vi "Add Vector Arrow to 3D Plot.vi"(6 "% of Shaft to Tip":dbl=0.8, 8 "Scale %":dbl=1.0, 9 "Unit Vector?":bool, 10 "Vector Color":u32(colorbox)=16879, 11 "Vector":dbl[](array[numeric])=[1.0, 0.0, 0.0]) -> (3 "Vector Arrow Object":refnum<vi>)   [LabVIEW 2010]
uses:
  <vilib>/picture/3D Picture Control/NI_3D Picture Control.lvlib
panel:
  out "3D Picture":refnum<vi>(3d-picture)
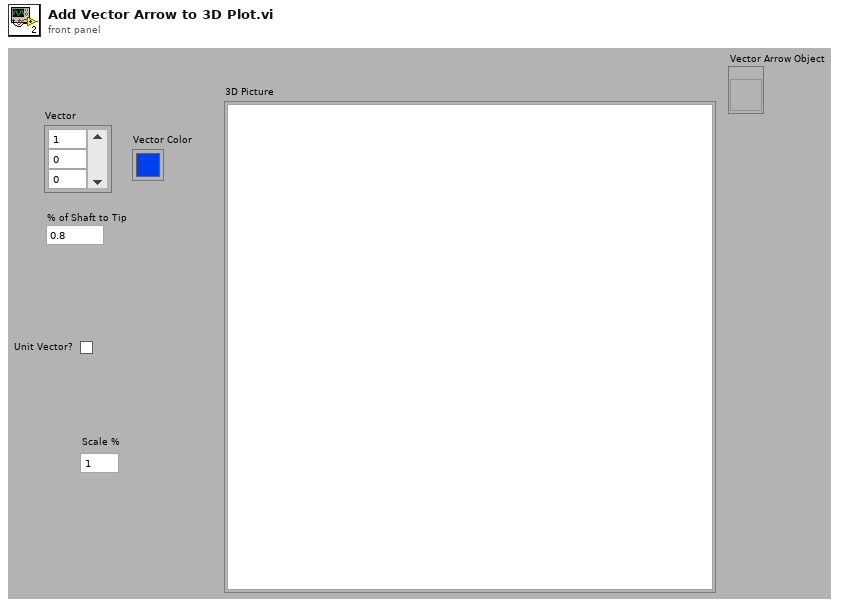
[diagram p1: front panel]
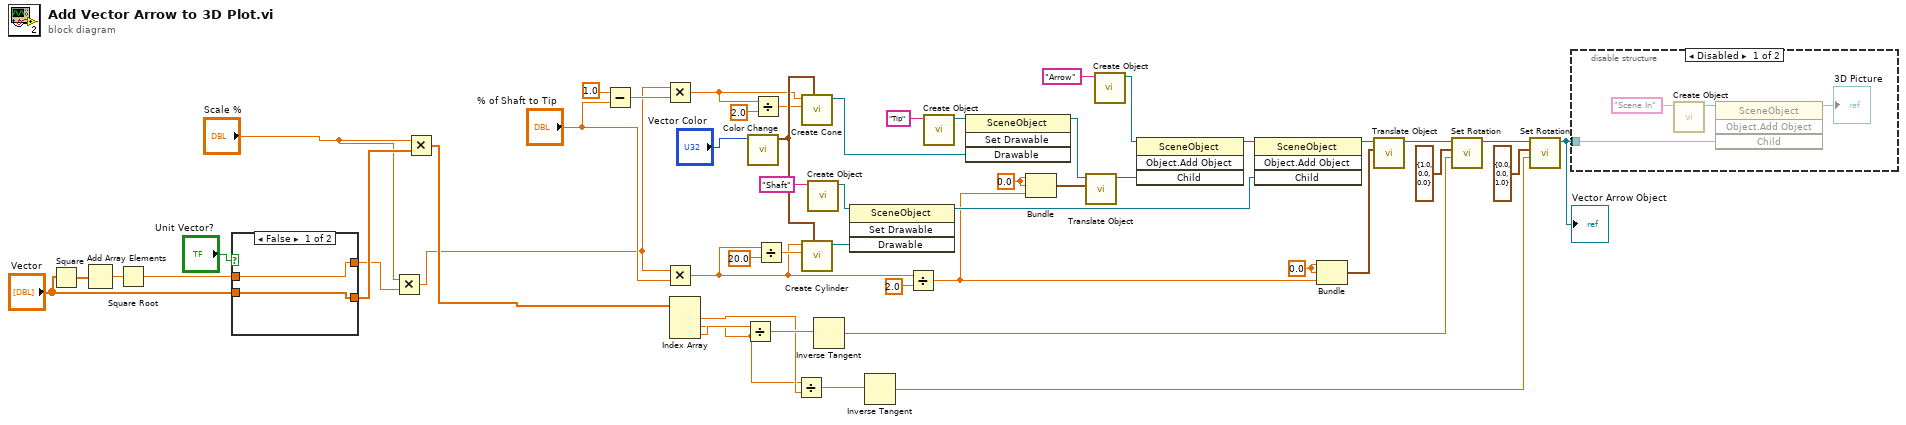
[diagram p0: block diagram]
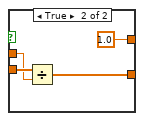
[diagram p2: hidden frame]
diagram:
  w23 = 0.0 ("x")
  w26 = 0.0 ("x")
  n1 = Square(x="Vector") -> (x^2=w20:dbl[])
  n2 = Add Array Elements(numeric array=w20) -> (sum=w19:dbl)
  n3 = Square Root(x=w19) -> (sqrt(x)=w16:dbl)
  n4 = case shown="False" "Unit Vector?" {
    tunnel: "Vector" -> [w53 w58]
    tunnel: w16 -> [w54 w57]
    tunnel: [w54 1.0] -> w3
    tunnel: [w53 w55] -> w5
    frame False {
    }
    frame True {
      n5 = Divide(x=w58, y=w57) -> (x/y=w55:dbl[])
    }
  }
  n6 = Multiply(x="Scale %", y=w3) -> (x*y=w1:dbl)
  n7 = Multiply(x="Scale %", y=w5) -> (x*y=w4:dbl[])
  n8 = Subtract(x=1.0, y="% of Shaft to Tip") -> (x-y=w38:dbl)
  n9 = Multiply(x=w1, y=w38) -> (x*y=w29:dbl)
  n10 = Multiply(x=w1, y="% of Shaft to Tip") -> (x*y=w30:dbl)
  n11 = Index Array(array=w4) -> (element #1=w8:dbl, element #2=w7:dbl, element #3=w12:dbl)  [unwired: 3 in]
  n12 = Divide(x=w12, y=w7) -> (x/y=w11:dbl)
  n13 = call <vilib>:"Color Change.vi"("Color"="Vector Color") -> ("RGBA"=w41:cluster{"R":sgl, "G":sgl, "B":sgl, "A":sgl})  [unwired: 10 in]
  n14 = Divide(x=w29, y=2.0) -> (x/y=w27:dbl)
  n15 = Divide(x=w30, y=20.0) -> (x/y=w31:dbl)
  n16 = Divide(x=w7, y=w8) -> (x/y=w9:dbl)
  n17 = call <vilib>:"Create Cone.vi"("Color"=w41, "Radius"=w27, "Height"=w29) -> ("New Cone Refnum"=w47:refnum<vi>)  [unwired: 7 in, 1 out]
  n18 = call <vilib>:"Create Cylinder.vi"("Color"=w41, "Radius"=w31, "Height"=w30) -> ("New Cylinder Refnum"=w46:refnum<vi>)  [unwired: 7 in, 1 out]
  n19 = call <vilib>:"Create Object.vi"("Name"="Shaft") -> ("Scene:New Object"=w44:refnum<vi>)  [unwired: 1 in, 9 out]
  n20 = Inverse Tangent(1:w11) -> (0:w10:dbl)
  n21 = invoke class="SceneObject" method="Set Drawable"(reference=w44, "Drawable"=w46) -> (reference out=w43:refnum<vi>)  [unwired: 2 in, 3 out]
  n22 = Inverse Tangent(1:w9) -> (0:w6:dbl)
  n23 = Divide(x=w30, y=2.0) -> (x/y=w21:dbl)
  n24 = call <vilib>:"Create Object.vi"("Name"="Tip") -> ("Scene:New Object"=w48:refnum<vi>)  [unwired: 1 in, 9 out]
  n25 = invoke class="SceneObject" method="Set Drawable"(reference=w48, "Drawable"=w47) -> (reference out=w37:refnum<vi>)  [unwired: 2 in, 3 out]
  n26 = Bundle("x"=w26, "x"=w26, w21) -> (w34:cluster{"x":dbl, "x":dbl, dbl})  [unwired: 1 in]
  n27 = call <vilib>:"Translate Object.vi"("Translation"=w34, "Scene.Object In"=w37) -> ("Scene.Object Out"=w36:refnum<vi>)  [unwired: 8 in, 1 out]
  n28 = call <vilib>:"Create Object.vi"("Name"="Arrow") -> ("Scene:New Object"=w51:refnum<vi>)  [unwired: 1 in, 9 out]
  n29 = invoke class="SceneObject" method="Object.Add Object"(reference=w51, "Child"=w36) -> (reference out=w50:refnum<vi>)  [unwired: 2 in, 3 out]
  n30 = invoke class="SceneObject" method="Object.Add Object"(reference=w50, "Child"=w43) -> (reference out=w25:refnum<vi>)  [unwired: 2 in, 3 out]
  n31 = Bundle("x"=w23, "x"=w23, w21) -> (w22:cluster{"x":dbl, "x":dbl, dbl})  [unwired: 1 in]
  n32 = call <vilib>:"Translate Object.vi"("Translation"=w22, "Scene.Object In"=w25) -> ("Scene.Object Out"=w24:refnum<vi>)  [unwired: 8 in, 1 out]
  n33 = call <vilib>:"Set Rotation.vi"("Angle"=w10, "Axis"=cluster{"X":sgl, "Y":sgl, "Z":sgl} {"X"=1.0, "Y"=0.0, "Z"=0.0}, "Scene Object"=w24) -> ("Rotated Scene Object"=w13:refnum<vi>)  [unwired: 7 in, 1 out]
  n34 = call <vilib>:"Set Rotation.vi"("Angle"=w6, "Axis"=cluster{"X":sgl, "Y":sgl, "Z":sgl} {"X"=0.0, "Y"=0.0, "Z"=1.0}, "Scene Object"=w13) -> ("Rotated Scene Object"=w33:refnum<vi>)  [unwired: 7 in, 1 out]
  "Vector Arrow Object" <- w33
  n35 = disable-structure shown="Disabled" {
    disable-tunnel: w33 -> [w59 _]
    frame Disabled {
      n36 = call <vilib>:"Create Object.vi"("Name"="Scene In") -> ("Scene:New Object"=w61:refnum<vi>)  [unwired: 1 in, 9 out]
      n37 = invoke class="SceneObject" method="Object.Add Object"(reference=w61, "Child"=w59) -> (reference out=→"3D Picture":refnum<vi>)  [unwired: 2 in, 3 out]
    }
    frame Enabled {
    }
  }
